vi "Error Query.vi"(0 "VISA Resource Name":refnum<visa-resource-name>, 11 "error in (no error)":errorcluster {"code" format="%.0x"}) -> (4 "VISA Resource Name Out":refnum<visa-resource-name>, 8 "Error":i32, 10 "Error Message":string, 15 "error out":errorcluster {"code" format="%.0x"})   [LabVIEW 2012, in "Agilent ESG Series.lvlib"]
doc: "This VI reads an error from the instrument. It expects to see errors in SCPI format (#,\"error message\"). If an error query is not supported, it returns a warning."
uses:
  Agilent ESG Series.lvlib
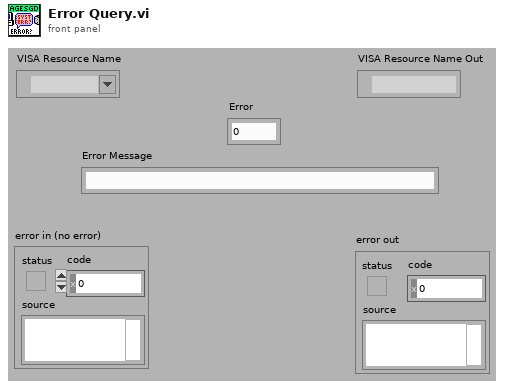
[diagram p1: front panel]
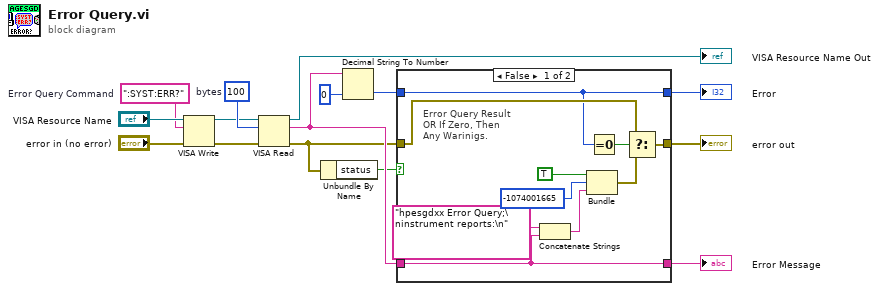
[diagram p0: block diagram]
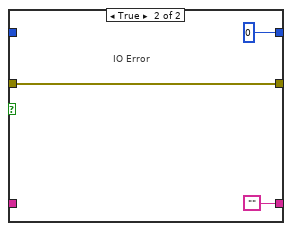
[diagram p2: hidden frame]
diagram:
  w11 = u32 100  # bytes
  w13 = ":SYST:ERR?"  # Error Query Command
  n1 = VISA Write(VISA resource name="VISA Resource Name", write buffer=w13, error in (no error)="error in (no error)") -> (VISA resource name out=w10:refnum<visa-resource-name>, error out=w12:errorcluster)  [unwired: 1 out]
  n2 = VISA Read(VISA resource name=w10, byte count=w11, error in (no error)=w12) -> (VISA resource name out=→"VISA Resource Name Out":refnum<visa-resource-name>, read buffer=w9:string, error out=w4:errorcluster)  [unwired: 1 out]
  n3 = Unbundle By Name(w4) -> ("status"=w8:bool)
  n4 = Decimal String To Number(string=w9, default (0L)=0) -> (number=w6:i32)  [unwired: 1 in, 1 out]
  n5 = case shown="False" w8 {
    tunnel: w9 -> [w23 _]
    tunnel: w4 -> [w19 w28]
    tunnel: [w20 w28] -> w2
    tunnel: [w23 ""] -> w1
    tunnel: [w16 0] -> w3
    tunnel: w6 -> [w16 _]
    frame False {
      # "Error Query Result\nOR If Zero, Then\nAny Warinigs."
      n6 = Concatenate Strings("hpesgdxx Error Query;\ninstrument reports:\n" ("Source"), w23) -> (w22:string)
      n7 = Bundle("Status"=TRUE, "Code"=-1074001665, w22) -> (w21:cluster{"Status":bool, "Code":i32, string})  [unwired: 1 in]
      n8 = Equal To 0?(x=w16) -> (x = 0?=w17:bool)
      n9 = Select(t=w19, s=w17, f=w21) -> (s? t:f=w20:errorcluster)
    }
    frame True {
      # "IO Error"
    }
  }
  "Error Message" <- w1
  "Error" <- w3
  "error out" <- w2
